vi "Configure Settling Delay.vi"(7 "Auto Settle (T: Enable)":bool=TRUE, 8 "error in (no error)":errorcluster, 10 "Manual Settling Delay (0 sec)":dbl, 11 "VISA resource name":refnum<visa-resource-name>) -> (0 "error out":errorcluster, 3 "VISA resource name out":refnum<visa-resource-name>)   [LabVIEW 2015, in "Keithley 24XX.lvlib"]
doc: "Configures the delay between the setting of the source and the taking of the measurement."
uses:
  <instrlib>/Keithley 24XX/Keithley 24XX.lvlib
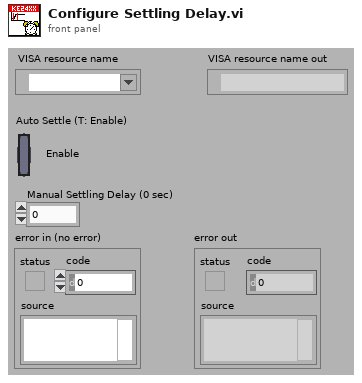
[diagram p1: front panel]
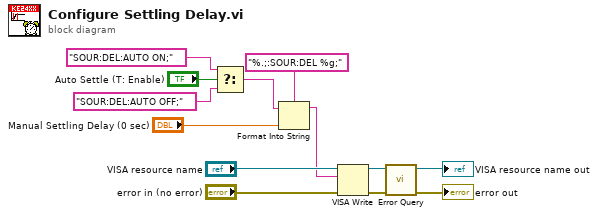
[diagram p0: block diagram]
diagram:
  n1 = Select(t="SOUR:DEL:AUTO ON;", s="Auto Settle (T: Enable)", f="SOUR:DEL:AUTO OFF;") -> (s? t:f=w4:string)
  n2 = Format Into String(format string="%.;:SOUR:DEL %g;", initial string=w4, "Manual Settling Delay (0 sec)") -> (resulting string=w1:string)  [unwired: 1 in, 1 out]
  n3 = VISA Write(VISA resource name="VISA resource name", write buffer=w1, error in (no error)="error in (no error)") -> (VISA resource name out=w8:refnum<visa-resource-name>, error out=w7:errorcluster)  [unwired: 1 out]
  n4 = call <instrlib>:"Error Query.vi"("error in (no error)"=w7, "VISA resource name"=w8) -> ("error out"=→"error out":errorcluster, "VISA resource name out"=→"VISA resource name out":refnum<visa-resource-name>)  [unwired: 6 in, 2 out]
